vi "controlReferenceAutoUpdate.vi"(7 "Set":bool, 8 "error in":errorcluster, 9 "ref auto up in":bool=TRUE, 10 "axis in":u8, 11 "connection ID":i32) -> (0 "error out":errorcluster, 1 "ref auto up out":bool=TRUE, 2 "axis out":u8, 3 "connection ID":i32)   [LabVIEW 2016]
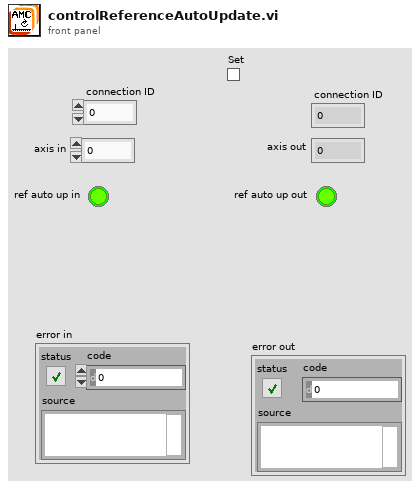
[diagram p1: front panel]
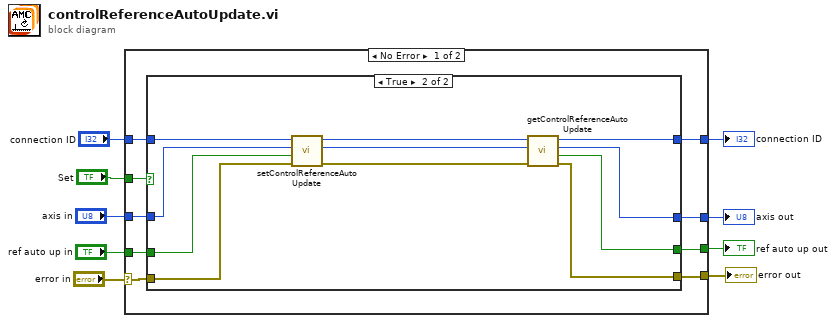
[diagram p0: block diagram]
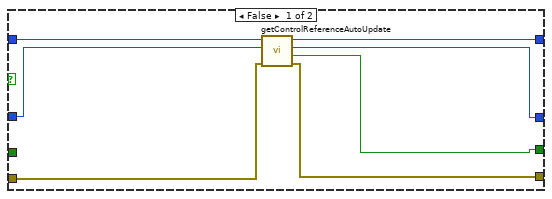
[diagram p2: hidden frame]
diagram:
  n1 = case shown="No Error" "error in" {
    selector: "error in" -> [w10 w40]
    tunnel: "axis in" -> [w16 w38]
    tunnel: [w11 w40] -> w8
    tunnel: [w13 w38] -> w7
    tunnel: "Set" -> [w17 _]
    tunnel: "ref auto up in" -> [w15 w39]
    tunnel: [w14 w37] -> w4
    tunnel: "connection ID" -> [w18 w37]
    tunnel: [w12 w39] -> w2
    frame No Error {
      n2 = case shown="True" w17 {
        tunnel: [w23 w28] -> w14
        tunnel: w18 -> [w24 w36]
        tunnel: w16 -> [w25 w35]
        tunnel: [w19 w29] -> w13
        tunnel: [w21 w31] -> w11
        tunnel: [w20 w30] -> w12
        tunnel: w15 -> [_ w33]
        tunnel: w10 -> [w22 w34]
        frame False {
          n3 = call "getControlReferenceAutoUpdate.vi"("error in"=w22, "axis"=w25, "connection ID"=w24) -> ("error out"=w21:errorcluster, "enabled"=w20:bool, "axis_out"=w19:i32, "connection ID"=w23:i32)  [unwired: 5 in]
        }
        frame True {
          n4 = call "setControlReferenceAutoUpdate.vi"("error in"=w34, "enable"=w33, "axis"=w35, "connection ID"=w36) -> ("error out"=w32:errorcluster, "axis_out"=w26:i32, "connection ID"=w27:i32)  [unwired: 5 in]
          n5 = call "getControlReferenceAutoUpdate.vi"("error in"=w32, "axis"=w26, "connection ID"=w27) -> ("error out"=w31:errorcluster, "enabled"=w30:bool, "axis_out"=w29:i32, "connection ID"=w28:i32)  [unwired: 5 in]
        }
      }
    }
    frame Error {
    }
  }
  "error out" <- w8
  "axis out" <- w7
  "ref auto up out" <- w2
  "connection ID" <- w4
